vi "Set Properties.vi"(5 "Property Values":variant[](array[variant]), 7 "Property Names":string[](array[string]), 8 "error in (no error)":errorcluster, 9 "Channel Name":string, 10 "Group Name":string, 11 "Data Logger Interface in":refnum<class "Data Logger Actor Interface.lvclass">) -> (0 "error out":errorcluster, 3 "Data Logger Interface out":refnum<class "Data Logger Actor Interface.lvclass">)   [LabVIEW 2024, in "Data Logger Actor Interface.lvlib" / "Data Logger Actor Interface.lvclass"]
uses:
  Data Logger Actor Interface.lvclass
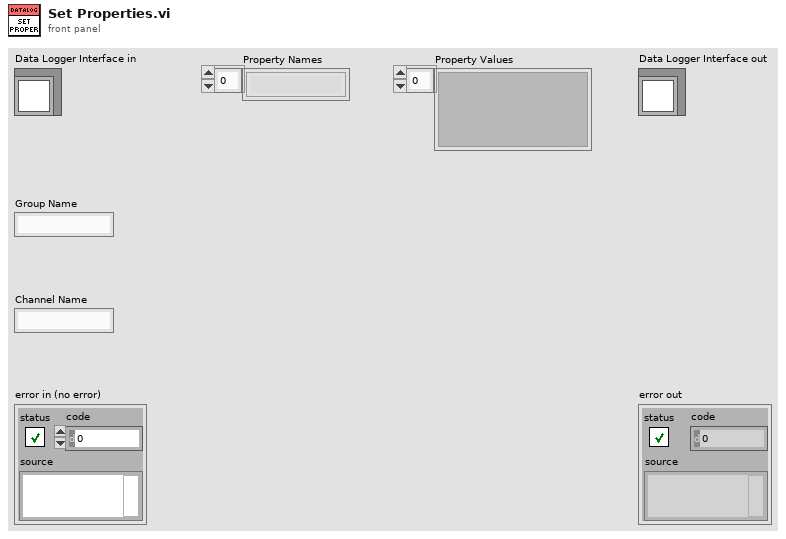
[diagram p1: front panel]
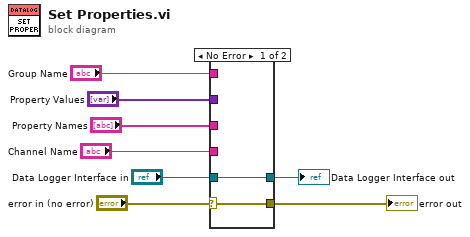
[diagram p0: block diagram]
diagram:
  n1 = case shown="No Error" "error in (no error)" {
    selector: "error in (no error)" -> [w9 w12]
    tunnel: [w9 w12] -> w7
    tunnel: [w10 w11] -> w5
    tunnel: "Data Logger Interface in" -> [w10 w11]
    tunnel: "Group Name" -> [_ _]
    tunnel: "Channel Name" -> [_ _]
    tunnel: "Property Names" -> [_ _]
    tunnel: "Property Values" -> [_ _]
    frame No Error {
    }
    frame Error {
    }
  }
  "error out" <- w7
  "Data Logger Interface out" <- w5
